vi "Raw_data_tweaker.vi"() -> ()   [LabVIEW 2010]
panel:
  in  "New Variable Value":string
  in  "Variable Name":string
  out "Files Processed":i32(slide) scale=0.0..8.0
  in  "stop":bool
  out "Current file being processed":path
  out "?":string[](array[string])
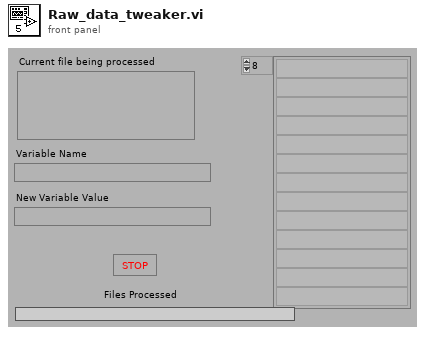
[diagram p1: front panel]
types:
  T1 = enum32{"existing file", "new file", "new or existing file", "existing dir", "new dir", "new or existing dir", "existing file (use LLBs)", "new file (use LLBs)", "new or existing file (use LLBs)", "new or existing file or directory (use LLBs)"}
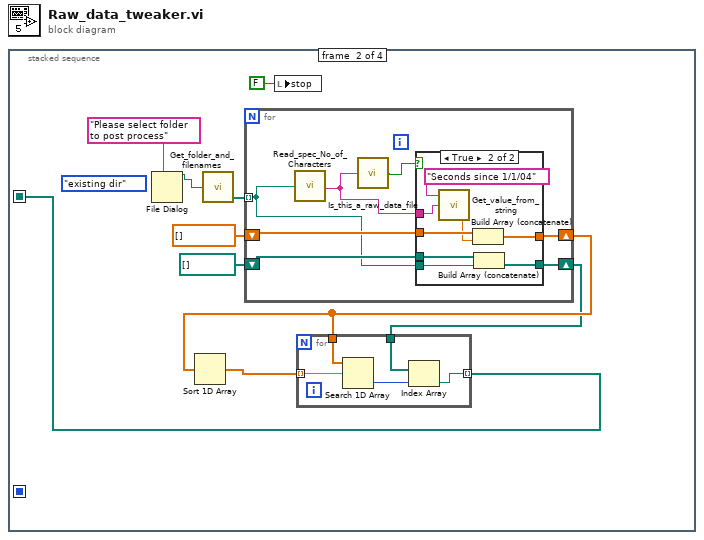
[diagram p0: block diagram]
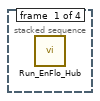
[diagram p2: hidden frame]
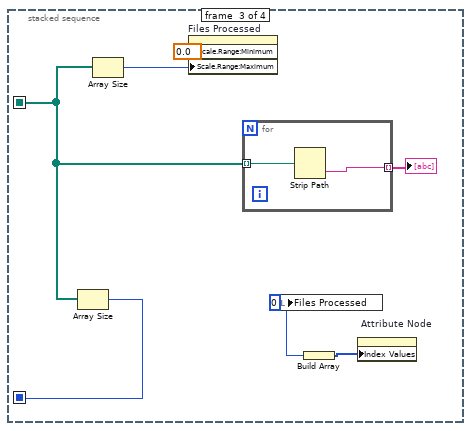
[diagram p4: hidden frame]
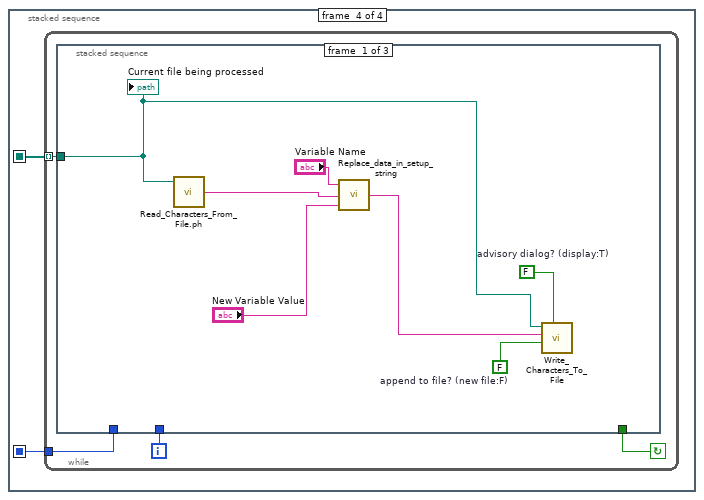
[diagram p5: hidden frame]
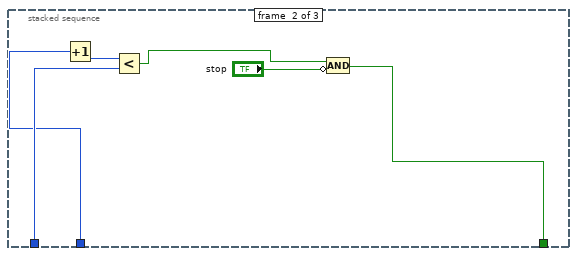
[diagram p6: hidden frame]
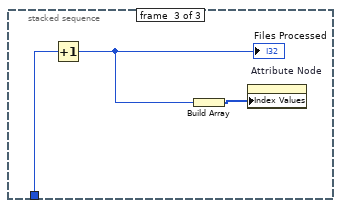
[diagram p7: hidden frame]
diagram:
  n1 = stacked-sequence {
    seq-local: [_ w2 _ _] -> [_ _ w37 w43]
    seq-local: [_ _ w38 _] -> [_ _ _ w42]
    frame #0 {
      n2 = call "Run_EnFlo_Hub.vi"() -> ()  [unwired: 8 in]
    }
    frame #1 {
      (unwired) T1."existing dir" ("select mode (2)")
      n3 = File Dialog(7:"Please select folder to post process" ("prompt")) -> (3:w3:path)  [unwired: 6 in, 3 out]
      n4 = call "Get_folder_and_filenames.vi"("file path (dialog if empty)"=w3) -> ("Files"=w5:path[])  [unwired: 1 out]
      n5 = for {
        tunnel: w5 -> [w16] mode=indexing
        shift-right: [w21] -> w9
        shift-left: dbl[] [] -> [w22]
        shift-right: [w19] -> w6
        shift-left: path[] [] -> [w20]
        n6 = call "Read_spec_No_of_Characters.vi"("Filename"=w16) -> ("character string"=w17:string)  [unwired: 1 out]
        n7 = call "Is_this_a_raw_data_file.vi"("character string"=w17) -> ("Raw Dat File?"=w18:bool)  [unwired: 2 in]
        n8 = case shown="True" w18 {
          tunnel: w22 -> [w24 w30]
          tunnel: [w24 w32] -> w21
          tunnel: w20 -> [w23 w28]
          tunnel: w16 -> [_ w27]
          tunnel: [w23 w26] -> w19
          tunnel: w17 -> [_ w25]
          frame False {
          }
          frame True {
            n9 = call "Get_value_from_string.vi"("Input string"=w25, "Variable name"="Seconds since 1/1/04") -> ("Value"=w29:dbl)  [unwired: 1 in, 1 out]
            n10 = Build Array (concatenate)(w30, w29) -> (w32:dbl[])
            n11 = Build Array (concatenate)(w28, w27) -> (w26:path[])
          }
        }
      }
      n12 = Sort 1D Array(array=w9) -> (sorted array=w8:dbl[])
      n13 = local write "stop"(FALSE ("stop")) -> ()
      n14 = for {
        tunnel: w9 -> [w15]
        tunnel: w8 -> [w14] mode=indexing
        tunnel: w6 -> [w13]
        tunnel: [w11] -> w2 mode=indexing
        n15 = Search 1D Array(1D array=w15, element=w14) -> (index of element=w12:i32)  [unwired: 1 in]
        n16 = Index Array(array=w13, index=w12) -> (element=w11:path)
      }
    }
    frame #2 {
      w33 = 0 ("Files Processed")
      n17 = Array Size(array=w37) -> (size(s)=w38:i32)
      n18 = Array Size(array=w37) -> (size(s)=w35:i32)
      n19 = property on="Files Processed" class="Slide (strict)"("Scale.Range:Minimum"=0.0 ("Write Attribute"), "Scale.Range:Maximum"=w35) -> ()  [unwired: 2 in, 2 out]
      n20 = for {
        tunnel: [w40] -> w39 mode=indexing
        tunnel: w37 -> [w41] mode=indexing
        n21 = Strip Path(path=w41) -> (name=w40:string)  [unwired: 1 out]
      }
      "?" <- w39
      n22 = local write "Files Processed"(w33) -> ()
      n23 = Build Array(w33) -> (w34:i32[])
      n24 = property on="Attribute Node" class="Arr (strict)"("Index Values"=w34) -> ()  [unwired: 2 in, 2 out]
    }
    frame #3 {
      n25 = while {
        tunnel: w42 -> [w46]
        tunnel: w43 -> [w47] mode=indexing
        i -> [w45]
        stop <- w44 continue-if-true
        n26 = stacked-sequence {
          tunnel: w47 -> [w49 _ _]
          tunnel: w46 -> [_ w57 _]
          tunnel: w45 -> [_ w56 w62]
          tunnel: [_ w55 _] -> w44
          frame #0 {
            w51 = FALSE  # append to file? (new file:F)
            w52 = FALSE  # advisory dialog? (display:T)
            n27 = call "Read_Characters_From_File.ph.vi"("file path (dialog if empty)"=w49) -> ("character string"=w48:string)  [unwired: 5 in, 3 out]
            n28 = call "Replace_data_in_setup_string.vi"("New data string"="New Variable Value", "Input string"=w48, "Variable name"="Variable Name") -> ("Appended string"=w50:string)
            n29 = call "Write_Characters_To_File.vi"("file path (dialog if empty)"=w49, "advisory dialog? (display:T)"=w52, "character string"=w50, "append to file? (new file:F)"=w51) -> ()  [unwired: 4 in, 1 out]
            "Current file being processed" <- w49
          }
          frame #1 {
            n30 = Increment(x=w56) -> (x+1=w60:i32)
            n31 = Less?(x=w60, y=w57) -> (x < y?=w58:bool)
            n32 = Compound Arithmetic op=AND(w58, invert "stop") -> (w55:bool)
          }
          frame #2 {
            n33 = Increment(x=w62) -> (x+1=w61:i32)
            "Files Processed" <- w61
            n34 = Build Array(w61) -> (w63:i32[])
            n35 = property on="Attribute Node" class="Arr (strict)"("Index Values"=w63) -> ()  [unwired: 2 in, 2 out]
          }
        }
      }
    }
  }
